vi "IN-0-OpAmp2.vi"() -> ()   [LabVIEW 2010]
panel:
  out "Rail -":bool
  out "Rail +":bool
  in  "Hi  Gain":bool
  out "Transfer Curve":cluster{dbl[], dbl[]}(graph)
  in  "Power":bool=TRUE
  out "Vout":dbl(knob) scale=-15.0..15.0 scale format="%.1f"
  in  "V+":dbl(slide) scale=-2.0..2.0 scale format="%.1f"
  in  "V-":dbl(slide) scale=-2.0..2.0 scale format="%.1f"
  # "[Press Run]"
  # "Vout = - (V- - V+)"
  # "Lo Gain"
  # "Vout"
  # "DV"
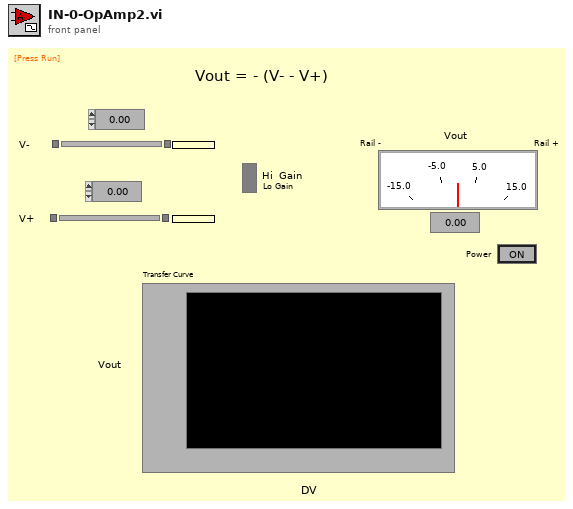
[diagram p1: front panel]
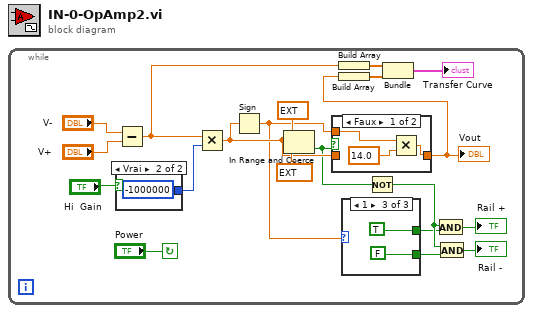
[diagram p0: block diagram]
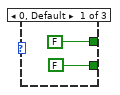
[diagram p2: hidden frame]
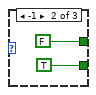
[diagram p3: hidden frame]
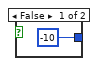
[diagram p4: hidden frame]
diagram:
  n1 = while {
    stop <- "Power" continue-if-true
    n2 = case shown="Vrai" "Hi  Gain" {
      tunnel: [-10 -1000000] -> w9
      frame False {
      }
      frame True {
      }
    }
    n3 = Subtract(x="V-", y="V+") -> (x-y=w14:dbl)
    n4 = Multiply(x=w14, y=w9) -> (x*y=w16:dbl)
    n5 = Sign(1:w16) -> (0:w2:dbl)
    n6 = In Range and Coerce(upper limit=ext 14.0 ("hi"), x=w16, lower limit=ext -14.0 ("lo")) -> (In Range?=w8:bool)  [unwired: 1 out]
    n7 = case shown="Faux" w8 {
      tunnel: w16 -> [_ w32]
      tunnel: [w30 w32] -> w11
      tunnel: w2 -> [w29 _]
      frame False {
        n8 = Multiply(x=w29, y=14.0) -> (x*y=w30:dbl)
      }
      frame True {
      }
    }
    "Vout" <- w11
    n9 = Build Array(w14) -> (w13:dbl[])
    n10 = Build Array(w11) -> (w12:dbl[])
    n11 = case shown="1" w2 {
      tunnel: [FALSE FALSE TRUE] -> w6
      tunnel: [FALSE TRUE FALSE] -> w5
      frame 0, Default {
      }
      frame -1 {
      }
      frame 1 {
      }
    }
    n12 = Not(x=w8) -> (.not. x?=w7:bool)
    n13 = Bundle(w13, w12) -> (→"Transfer Curve":cluster{dbl[], dbl[]})  [unwired: 1 in]
    n14 = And(x=w7, y=w6) -> (x .and. y?=→"Rail +":bool)
    n15 = And(x=w7, y=w5) -> (x .and. y?=→"Rail -":bool)
  }
